vi "New.vi"(8 "error in (no error)":errorcluster, 9 "command":refnum<k21>, 10 "property":refnum<k21>) -> (0 "error out":errorcluster, 3 "DevicePropertyRelay out":refnum<class "DevicePropertyRelay.lvclass">)   [LabVIEW 2015, in "DevicePropertyRelay.lvclass"]
uses:
  DevicePropertyRelay.lvclass
  DevicePropertyRelay.lvclass/DevicePropertyRelay.ctl
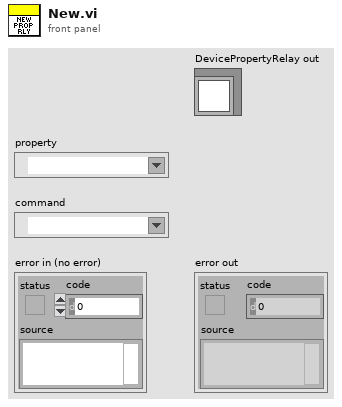
[diagram p1: front panel]
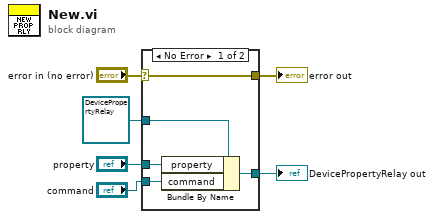
[diagram p0: block diagram]
diagram:
  n1 = case shown="No Error" "error in (no error)" {
    selector: "error in (no error)" -> [w11 w13]
    tunnel: [w11 w13] -> w5
    tunnel: [w9 w12] -> w3
    tunnel: refnum<class "DevicePropertyRelay.lvclass"> refnum ("DevicePropertyRelay in") -> [w10 w12]
    tunnel: "property" -> [w8 _]
    tunnel: "command" -> [w7 _]
    frame No Error {
      n2 = Bundle By Name(cluster=w10, "property"=w8, "command"=w7) -> (w9:refnum<class "DevicePropertyRelay.lvclass">)
    }
    frame Error {
    }
  }
  "error out" <- w5
  "DevicePropertyRelay out" <- w3
